vi "RSNRPZ Set ContAv Smoothing State.vi"(8 "error in (no error)":errorcluster, 9 "ContAv Smoothing (T: On)":bool=TRUE, 10 "Channel (1)":i32=1, 11 "VISA session":refnum<visa-resource-name> caption="VISA resource name") -> (0 "error out":errorcluster, 3 "dup VISA session":refnum<visa-resource-name> caption="VISA resource name")   [LabVIEW 2019]
doc: "This VI activates digital lowpass filtering of the sampled video signal.\nThe problem of instable display values due to a modulation of a test signal can also be eliminated by lowpass filtering of the video signal. The lowpass filter eliminates the variations of the display even in case of unperiodic modulation and does not require any other setting.\nIf the modulation is periodic, the setting of the sampling window is the better method since it allows for shorter measurement times.\n\nRemote-control command(s):\nSENS:POW:AVG:SMO:STAT ON | OFF"
uses:
  rsnrpz_32.dll
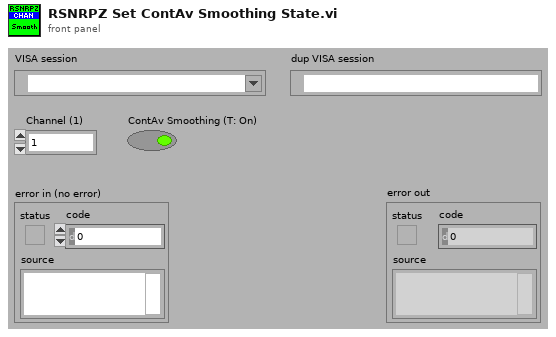
[diagram p1: front panel]
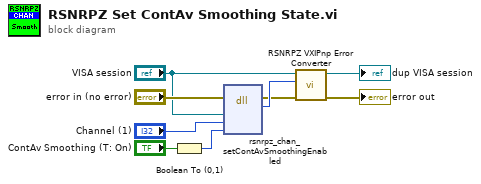
[diagram p0: block diagram]
diagram:
  n1 = Boolean To (0,1)(Boolean="ContAv Smoothing (T: On)") -> (0, 1=w6:i16)
  n2 = dll-call lib="C:/Users/LABadmin/Documents/Jarvis/user_lib/rsnrpz/rsnrpz_32.dll" fn="rsnrpz_chan_setContAvSmoothingEnabled"(error in="error in (no error)", "VISA Session"="VISA session", "Channel"="Channel (1)", "ContAv Smoothing"=w6) -> (error out=w5:errorcluster, "Status"=w8:i32)  [unwired: 5 in, 1 out]
  n3 = call <instrlib>:"RSNRPZ VXIPnp Error Converter.vi"("error in"=w5, "VXIPnp error code"=w8, "VISA session"="VISA session") -> ("error out"=→"error out":errorcluster, "dup VISA session"=→"dup VISA session":refnum<visa-resource-name>)  [unwired: 7 in]
